vi "CloseSensor.vi"(0 "Fehler (Eingang, kein Fehler)":errorcluster, 5 "instanceHandle":u32, 7 "DLL-Path":path) -> (4 "Fehler (Ausgang)":errorcluster, 6 "instanceHandle":u32, 8 "DLL-Path":path, 10 "ERR_CODE":i32)   [LabVIEW 2015, in "MEDAQLib.lvlib"]
doc: "ERR_CODE CloseSensor (DWORD instanceHandle);\n\nClose the connection to the sensor."
uses:
  MEDAQLib.lvlib
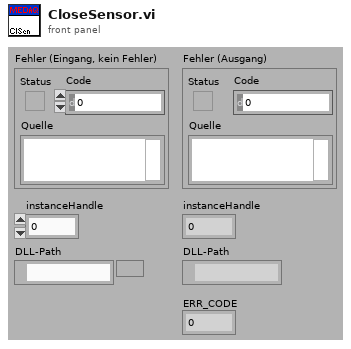
[diagram p1: front panel]
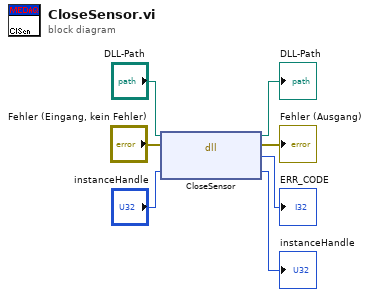
[diagram p0: block diagram]
diagram:
  n1 = dll-call lib="C:/Programme/National Instruments 8.6/LabVIEW 8.6/instr.lib/MEDAQLib/Release/MEDAQLib.dll" fn="CloseSensor"(path in="DLL-Path", error in="Fehler (Eingang, kein Fehler)", "instanceHandle"="instanceHandle") -> (path out=→"DLL-Path":path, error out=→"Fehler (Ausgang)":errorcluster, "Rückgabetyp"=→"ERR_CODE":i32, "instanceHandle"=→"instanceHandle":u32)  [unwired: 1 in]
